vi "SaveAcqData I8.vi"(0 "File Name":string, 2 "Header In":string, 3 "Array":i8[][](array[numeric]), 4 "Ext":string=".tmp", 5 "Use Input Header?":bool) -> ()   [LabVIEW 2022 SP3]
uses:
  ScanningControl/Motion Controllers/-MotionRoutines/MotionGlobals.vi
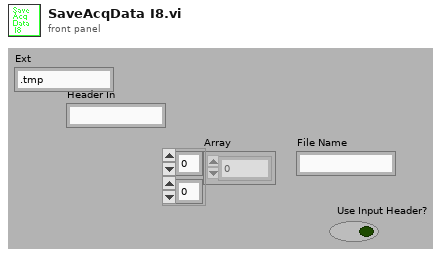
[diagram p1: front panel]
types:
  T1 = enum16{"open", "replace", "create", "open or create", "replace or create", "replace or create with confirmation"}
  T2 = enum16{"deny read/write", "deny write-only", "deny none"}
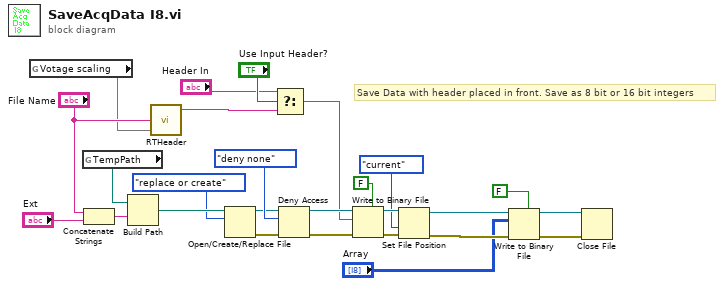
[diagram p0: block diagram]
diagram:
  # "Save Data with header placed in front. Save as 8 bit or 16 bit integers"
  n1 = global read "MotionGlobals.vi" "Votage scaling"() -> (w4)
  n2 = global read "MotionGlobals.vi" "TempPath"() -> (w26:path)
  n3 = Concatenate Strings("File Name", "Ext") -> (w25:string)
  n4 = Build Path(base path=w26, name or relative path=w25) -> (appended path=w24:path)
  n5 = call "RTHeader.vi"("File Name In"="File Name", "Votage scaling"=w4) -> ("Header String Out"=w6:string)  [unwired: 4 in, 1 out]
  n6 = Open/Create/Replace File(file path (use dialog)=w24, operation (0:open)=T1."replace or create") -> (refnum out=w19:refnum<file>, error out=w20:errorcluster)  [unwired: 1 in, 4 out]
  n7 = Select(t="Header In", s="Use Input Header?", f=w6) -> (s? t:f=w7:string)
  n8 = Deny Access(4:w20, 6:T2."deny none" ("deny mode (2)"), 7:w19) -> (0:w22:errorcluster, 3:w23:refnum<file>)
  n9 = Write to Binary File(file (use dialog)=w23, data=w7, error in=w22, 5:FALSE ("prepend array or string size? (T)")) -> (refnum out=w16:refnum<file>, error out=w15:errorcluster)  [unwired: 3 out]
  n10 = Set File Position(refnum=w16, from (0:start)=enum16{"start", "end", "current"}."current" ("pos mode (0:2)"), error in=w15) -> (refnum out=w13:refnum<file>, error out=w12:errorcluster)  [unwired: 1 out]
  n11 = Write to Binary File(file (use dialog)=w13, data="Array", error in=w12, 5:FALSE) -> (refnum out=w11:refnum<file>, error out=w10:errorcluster)  [unwired: 1 in, 2 out]
  n12 = Close File(refnum=w11, error in=w10) -> ()  [unwired: 2 out]
